vi "Event Handler.vi"(0 "Tamer in":refnum<class "Tamer.lvclass">, 5 "Event type":T1=enum."Message", 7 "Item Name":string, 9 "Data":variant, 11 "error in (no error)":errorcluster) -> (4 "Tamer out":refnum<class "Tamer.lvclass">, 15 "error out":errorcluster)   [LabVIEW 2020, in "Tamer.lvlib" / "Tamer.lvclass"]
doc: "This VI is the event handler of the uService: every time an event is triggered to the uService, this VI is called.\nNote: here you can access the Actor/Class data, but it will be the one coming out from Init. You cannot modify the values.\nThree different events are supported:\nI) Button Pressed: get called on a GUI button pressed. Item Name is the name (label) of the button, Data is empty.\nII) Shared Variable Updated: get called when a SV you subscribed to is updated. Item Name is the name of the SV, and Data is the value (note: you need to convert it to the proper type).\nIII) Message: get called every time a user event is generated using Send Message to Event Handler. The values of Item Name and Data are the one given to the Send Message to Event Handler.\nIV) Ready to launch?: this frame get called every time a new Run is initiated. Each uService is responsible of performing a self check before giving back the green light for the Run to start."
uses:
  Tamer.lvclass
  C:/Users/marco/Documents/GitHub_Lab/TALOS/talos/Father of all uServices/Father of all uServices/Father of all uServices.lvclass
  Father of all uServices/Father of all uServices/Event Handler Items.ctl
  Ancestor/Ancestor/Ancestor.lvclass/Ancestor.ctl
  Tamer Consumer Case Selector.ctl
  Father of all uServices/Father of all uServices Messages/Consumer Msg/Consumer Msg.lvclass/Consumer Msg.ctl
  Support VIs/Go-NoGo.ctl
  Run Utilities/TypeDefs/Messages/Monkey Status Message.ctl
  Run Utilities/TypeDefs/Monkey Status.ctl
  Run Utilities/Schedule/Schedule.lvclass
  Run Utilities/TypeDefs/Messages/Script Checker Message.ctl
  Run Utilities/TypeDefs/Script Checker Result.ctl
  Run Utilities/TypeDefs/Messages/Banana Message.ctl
  Run Utilities/TypeDefs/Return Code.ctl
  Guardian/Guardian Messages/Message to uService Msg/Message to uService Msg.lvclass/Message to uService Msg.ctl
  Tamer.lvclass/Tamer.ctl
  Guardian/Guardian/Requests.ctl
  Guardian/Guardian Messages/Requests from uServices Msg/Requests from uServices Msg.lvclass/Requests from uServices Msg.ctl
  FGV/Error Memory/Get Error Description.vi
  Support VIs/Get PC name.vi
  Ancestor/Ancestor/Read ID.vi
  Support VIs/Get Class Name.vi
  <vilib>/Utility/error.llb/Clear Errors.vi
  Father of all uServices/Father of all uServices Messages/Consumer Msg/Send Consumer.vi
  Guardian/Guardian Messages/Message to uService Msg/Send Message to uService.vi
  Guardian/Guardian Messages/Requests from uServices Msg/Send Requests from uServices.vi
  FGV/Error Memory/Error Memory Core.vi
  <vilib>/AdvancedString/Delimited String to 1D String Array.vi
  Support VIs/Circus Root Path.vi
  FGV/Error Memory/Error Crt Lvl checker.vi
  FGV/Error Memory/Error Memory Core.vi/40c8088d-b597-4017-91af-faa98e00292e.vi
  FGV/Error Memory/Error Memory Core.vi/d4a3ab98-063c-4e44-b43d-fbdcfe6c2be2.vi
  Father of all uServices/Father of all uServices/Father of all uServices.lvclass
  C:/Users/marco/Documents/GitHub_Lab/TALOS/builds/Actor Framework PPL/Actor Framework.lvlibp/1abvi3w/vi.lib/ActorFramework/Actor/Actor.lvclass
  Support VIs/Global Memory.vi
  <vilib>/Utility/LVClass/Get LV Class Name.vi
  Support VIs/Is in Packed Library.vi
  Support VIs/TALOS Root path.vi
  Support VIs/Read CSV worksheet.vi
  Support VIs/Global Constants.vi
  <vilib>/Utility/error.llb/General Error Handler.vi
  builds/Actor Framework PPL/Actor Framework.lvlibp/1abvi3w/vi.lib/ActorFramework/Actor/Read Self Enqueuer.vi
  <userlib>/_OpenG.lib/lvdata/lvdata.llb/Get Strings from Enum__ogtk.vi
  builds/Actor Framework PPL/Actor Framework.lvlibp/1abvi3w/vi.lib/ActorFramework/Message Enqueuer/Enqueue.vi
  Support VIs/Error Log.vi
  Open Debug Window.vi
  builds/Actor Framework PPL/Actor Framework.lvlibp/1abvi3w/vi.lib/ActorFramework/Actor/Read Caller Enqueuer.vi
  Ancestor/Ancestor/Ancestor.lvclass
  <vilib>/Comparison/Equal/Equal Functor/Equal Functor.lvclass
  Father of all uServices/Father of all uServices Messages/Consumer Msg/Consumer Msg.lvclass
  Guardian/Guardian Messages/Message to uService Msg/Message to uService Msg.lvclass
  Guardian/Guardian Messages/Requests from uServices Msg/Requests from uServices Msg.lvclass
  TALOS.lvlib
  Guardian/Guardian/Guardian.lvclass
  Run Utilities/Run Utilities.lvlib
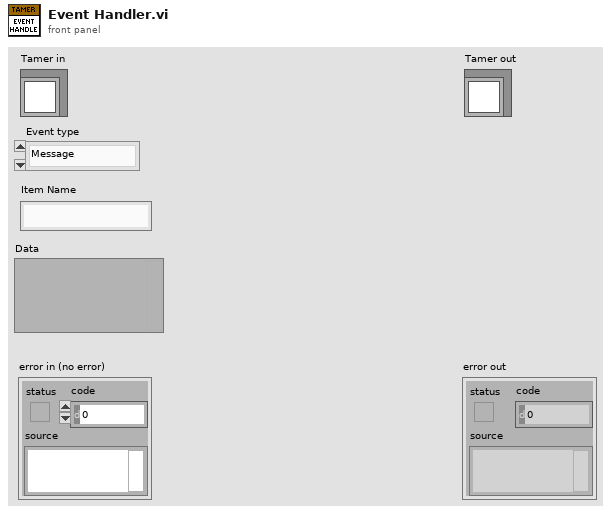
[diagram p1: front panel]
types:
  T1 = typedef "TALOS.lvlib/Father of all uServices.lvlib/Father of all uServices.lvclass/Event Handler Items.ctl" = enum16{"Button Pressed", "Shared Variable Updated", "Message", "Ready to launch?", "Safe Mode", "Start RUN", "Stop RUN"}
  T2 = typedef "Tamer.lvlib/Tamer.lvclass/Tamer Consumer Case Selector.ctl" = enum16{"New schedule", "Initiate RUN", "Parse Schedules", "Script Checker", "Banana after Quality Check", "Update Crit Lvl", "Propagate Banana", "Reply from Guardian", "Reply from uService", "Timeout of RUN", "uService Replies Check", "Update from Monkey", "Monkey Died", "Reschedule", "Rerun", "Stop DAQ", "Stop Schedule", "Skip Run", "Kill Process", "Update GV"}
  T3 = enum32{"Invalid", "Standard", "Closed", "Hidden", "Minimized", "Maximized"}
  T4 = typedef "TALOS.lvlib/Go-NoGo.ctl" = cluster{"ID":string, "Status":bool, "Data":string[], "GUID":string}
  T5 = typedef "TALOS.lvlib/Run Utilities.lvlib/Monkey Status Message.ctl" = cluster{"Monkey ID":string, "Monkey Status":T6, "Scripts left":u32, "ETA":string, "Current Action":string, "Report from previous RUNs":string, "Skipped RUNs":refnum<class "Schedule.lvclass">}
  T6 = typedef "TALOS.lvlib/Run Utilities.lvlib/Monkey Status.ctl" = enum16{"Init", "Paused", "Ongoing", "Stopped", "Finished (no errors)", "Finished (with errors)"}
  T7 = typedef "TALOS.lvlib/Run Utilities.lvlib/Script Checker Message.ctl" = cluster{"Monkey ID":string, "Script Checker Result":T8}
  T8 = typedef "TALOS.lvlib/Run Utilities.lvlib/Script Checker Result.ctl" = enum16{"Passed", "Failed", "Empty"}
  T9 = typedef "TALOS.lvlib/Run Utilities.lvlib/Return Code.ctl" = enum16{"All Good", "Retry", "Skip", "Skip All", "ABORT"}
  T10 = typedef "TALOS.lvlib/Run Utilities.lvlib/Banana Message.ctl" = cluster{"FPGA Name":string, "Return Code":T9}
  T11 = typedef "TALOS.lvlib/Guardian.lvlib/Guardian.lvclass/Requests.ctl" = enum16{"Ready to Launch", "Start RUN", "Stop RUN", "Update DAQ Params", "Update Error Listbox", "Update Run Status", "Update Kasli Log", "Run Stopped with Errors", "Switch uS View"}
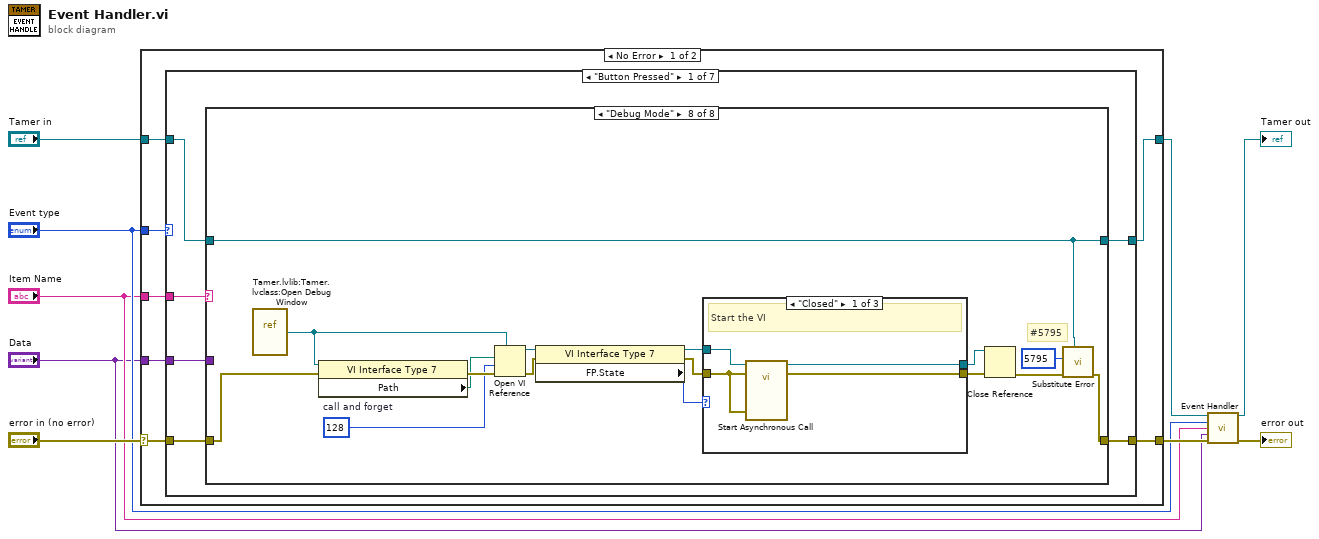
[diagram p0: block diagram]
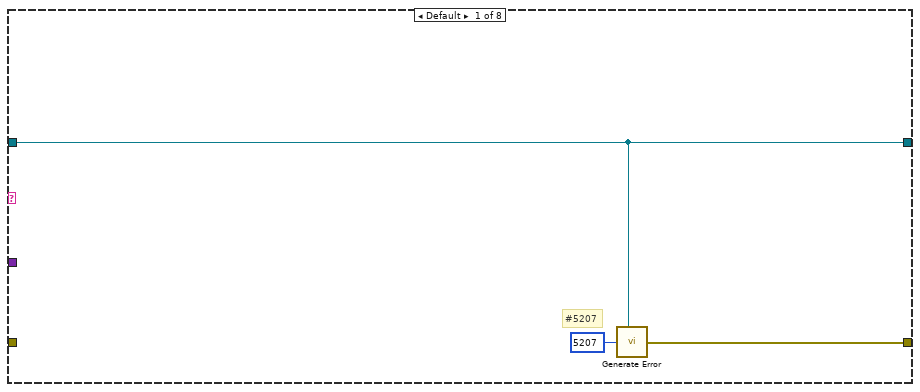
[diagram p2: hidden frame]
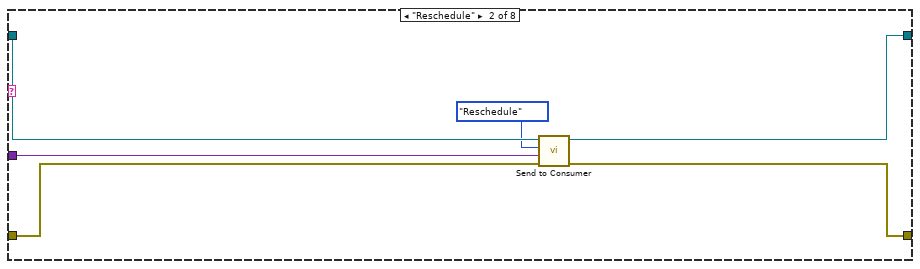
[diagram p3: hidden frame]
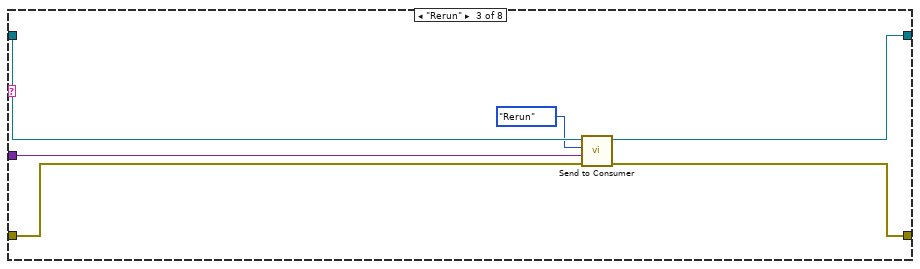
[diagram p4: hidden frame]
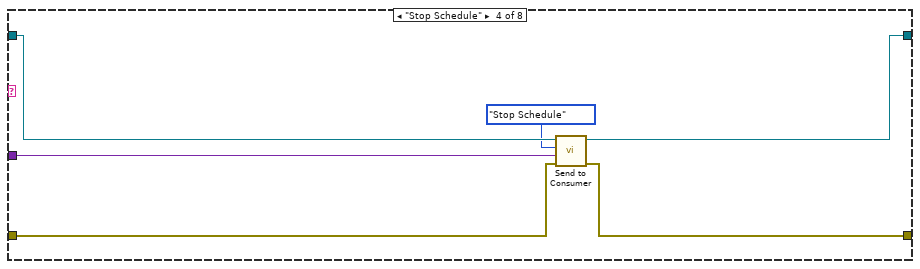
[diagram p5: hidden frame]
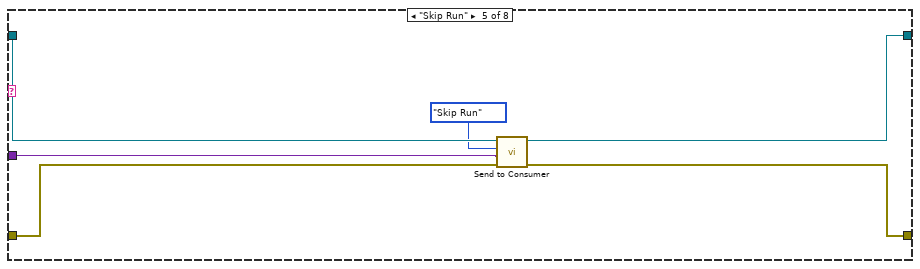
[diagram p6: hidden frame]
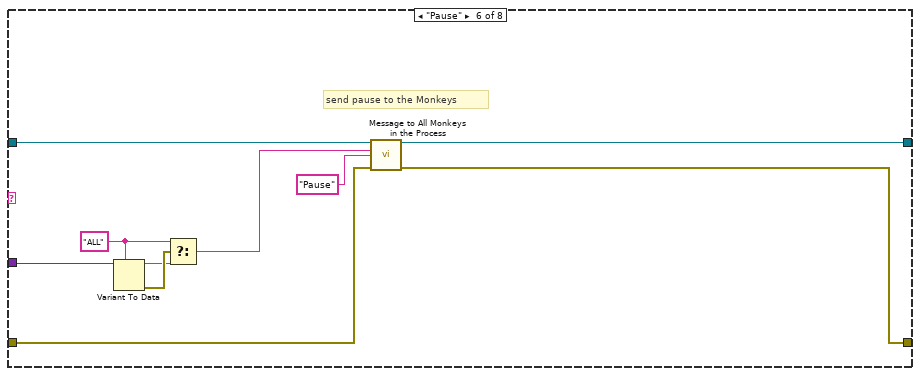
[diagram p7: hidden frame]
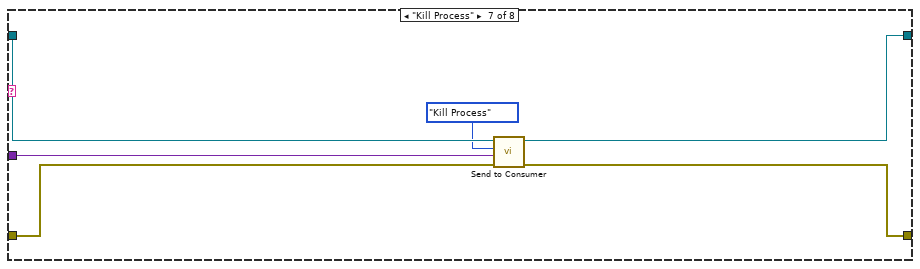
[diagram p8: hidden frame]
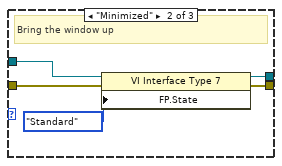
[diagram p9: hidden frame]
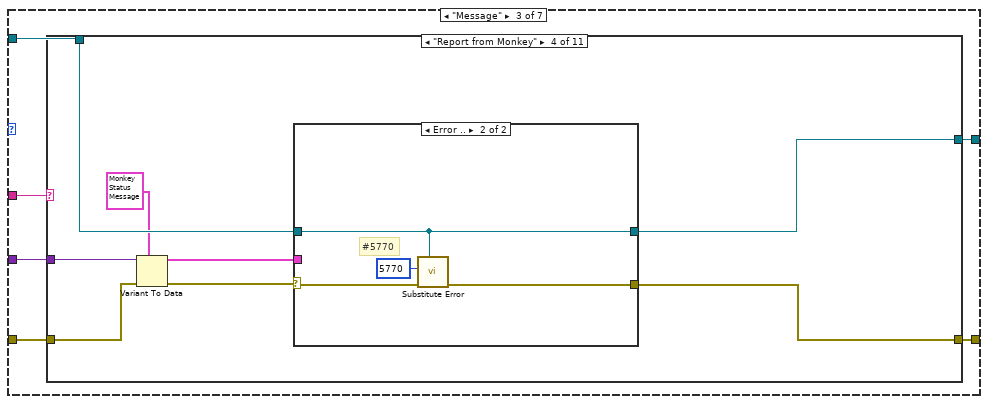
[diagram p12: hidden frame]
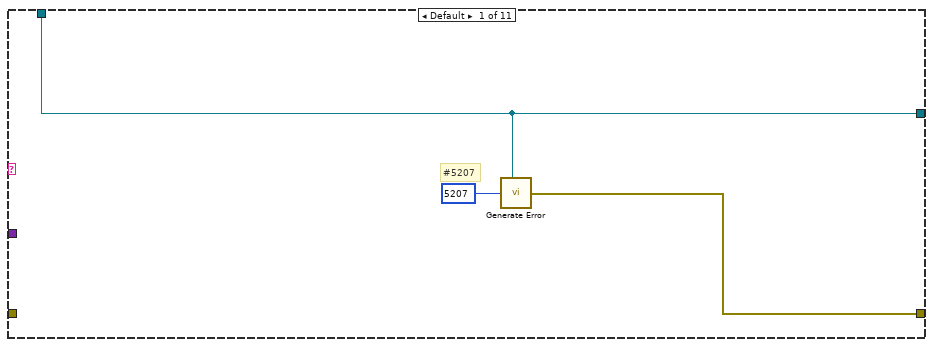
[diagram p13: hidden frame]
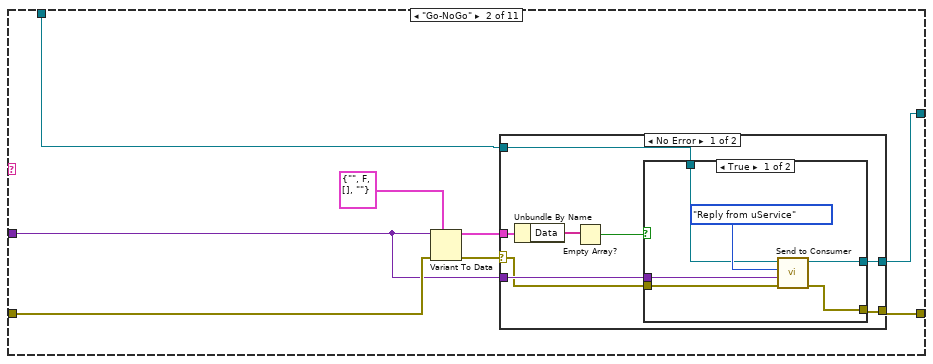
[diagram p14: hidden frame]
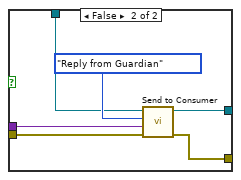
[diagram p15: hidden frame]
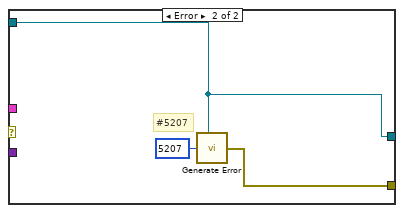
[diagram p16: hidden frame]
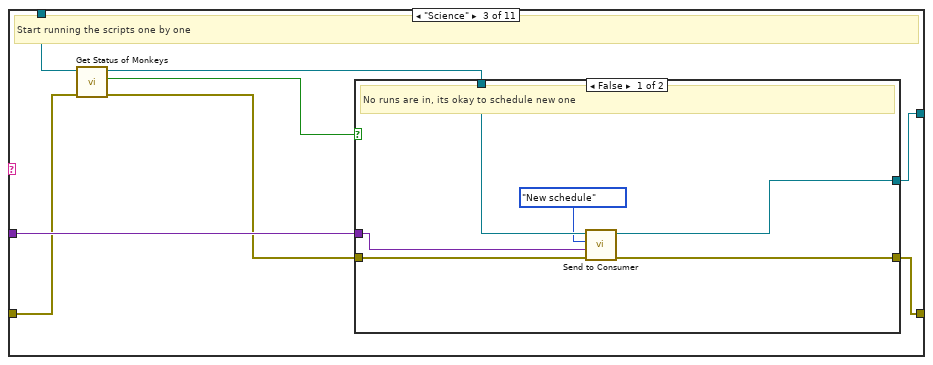
[diagram p17: hidden frame]
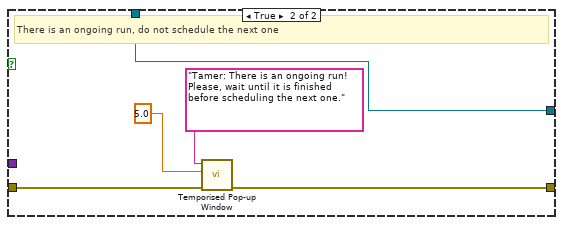
[diagram p18: hidden frame]
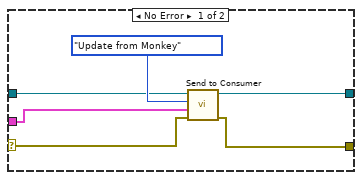
[diagram p19: hidden frame]
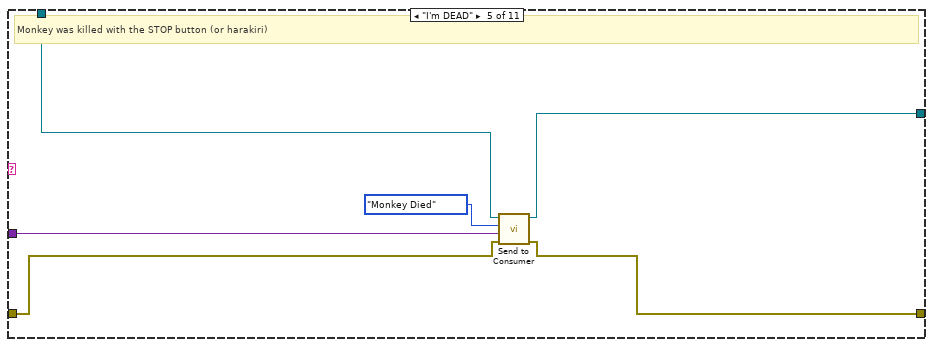
[diagram p20: hidden frame]
diagram:
  n1 = case shown="No Error" "error in (no error)" {
    selector: "error in (no error)" -> [w14 w330]
    tunnel: [w15 w330] -> w7
    tunnel: [w11 w329] -> w4
    tunnel: "Tamer in" -> [w10 w329]
    tunnel: "Event type" -> [w16 _]
    tunnel: "Item Name" -> [w13 _]
    tunnel: "Data" -> [w12 _]
    frame No Error {
      n2 = case shown="\"Button Pressed\"" w16 {
        tunnel: [w22 w94 w96 w307 w316 w321 w328] -> w15
        tunnel: w14 -> [w19 w94 w100 w308 w318 w322 w326]
        tunnel: w13 -> [w20 _ w99 _ _ _ _]
        tunnel: w10 -> [w21 w93 w97 w306 w313 w323 w327]
        tunnel: w12 -> [w17 _ w98 w304 _ _ _]
        tunnel: [w18 w93 w95 w303 w315 w319 w324] -> w11
        frame "Button Pressed" {
          n3 = case shown="\"Debug Mode\"" w20 {
            tunnel: w19 -> [_ w26 w32 w39 w45 w56 w63 w77]
            tunnel: [w24 w30 w35 w42 w46 w55 w60 w66] -> w22
            tunnel: w21 -> [w23 w31 w37 w43 w49 w58 w65 w67]
            tunnel: [w23 w28 w34 w41 w47 w57 w61 w67] -> w18
            tunnel: w17 -> [_ w27 w33 w38 w44 w54 w62 _]
            frame Default {
              # "#5207"
              n4 = call "Generate Error.vi"("Class"=w23, "Error Code"=5207) -> ("error out"=w24:errorcluster)  [unwired: 5 in]
            }
            frame "Reschedule" {
              n5 = call "Send to Consumer.vi"("error in (no error)"=w26, "Data"=w27, "Case ID"=Tamer_Consumer_Case_Selector."Reschedule" ("Monkey Consumer Case Selector"), "uService Template in"=w31) -> ("error out"=w30:errorcluster, "uService Template out"=w28:refnum<class "Tamer.lvclass">)  [unwired: 6 in]
            }
            frame "Rerun" {
              n6 = call "Send to Consumer.vi"("error in (no error)"=w32, "Data"=w33, "Case ID"=Tamer_Consumer_Case_Selector."Rerun" ("Monkey Consumer Case Selector"), "uService Template in"=w37) -> ("error out"=w35:errorcluster, "uService Template out"=w34:refnum<class "Tamer.lvclass">)  [unwired: 6 in]
            }
            frame "Stop Schedule" {
              n7 = call "Send to Consumer.vi"("error in (no error)"=w39, "Data"=w38, "Case ID"=Tamer_Consumer_Case_Selector."Stop Schedule" ("Monkey Consumer Case Selector"), "uService Template in"=w43) -> ("error out"=w42:errorcluster, "uService Template out"=w41:refnum<class "Tamer.lvclass">)  [unwired: 6 in]
            }
            frame "Skip Run" {
              n8 = call "Send to Consumer.vi"("error in (no error)"=w45, "Data"=w44, "Case ID"=Tamer_Consumer_Case_Selector."Skip Run" ("Monkey Consumer Case Selector"), "uService Template in"=w49) -> ("error out"=w46:errorcluster, "uService Template out"=w47:refnum<class "Tamer.lvclass">)  [unwired: 6 in]
            }
            frame "Pause" {
              w53 = "ALL"
              # "send pause to the Monkeys"
              n9 = Variant To Data(type=w53, Variant=w54) -> (data=w52:string, error out=w59:errorcluster)  [unwired: 1 in]
              n10 = Select(t=w53, s=w59, f=w52) -> (s? t:f=w51:string)
              n11 = call-dynamic "Message to All Monkeys in the Process.vi"("Tamer in"=w58, "Process ID"=w51, "Message"="Pause" ("Process ID"), "error in (no error)"=w56) -> ("Tamer out"=w57:refnum<class "Tamer.lvclass">, "error out"=w55:errorcluster)  [unwired: 10 in]
            }
            frame "Kill Process" {
              n12 = call "Send to Consumer.vi"("error in (no error)"=w63, "Data"=w62, "Case ID"=Tamer_Consumer_Case_Selector."Kill Process" ("Monkey Consumer Case Selector"), "uService Template in"=w65) -> ("error out"=w60:errorcluster, "uService Template out"=w61:refnum<class "Tamer.lvclass">)  [unwired: 6 in]
            }
            frame "Debug Mode" {
              w78 = 128  # call and forget
              # "#5795"
              n13 = vi-ref "Tamer.lvlib:Tamer.lvclass:Open Debug Window.vi"() -> (w76:refnum<vi>)
              n14 = property class="VI Interface Type 7"(reference=w76, error in=w77) -> (error out=w81:errorcluster, "Path"=w80:path)  [unwired: 1 out]
              n15 = Open VI Reference(type specifier VI Refnum (for type only)=w76, vi path=w80, options=w78, error in (no error)=w81) -> (vi reference=w79:refnum<vi>, error out=w74:errorcluster)  [unwired: 2 in]
              n16 = property class="VI Interface Type 7"(reference=w79, error in=w74) -> (reference out=w75:refnum<vi>, error out=w73:errorcluster, "FP.State"=w72:T3)
              n17 = case shown="\"Closed\"" w72 {
                tunnel: w75 -> [w85 w88 w92]
                tunnel: w73 -> [w84 w90 w91]
                tunnel: [w83 w89 w91] -> w69
                tunnel: [w82 w86 w92] -> w68
                frame "Closed" {
                  # "Start the VI"
                  n18 = call-by-ref "Start Asynchronous Call"(reference=w85, error in=w84, 8:"error in (no error)"=w84) -> (reference out=w82:refnum<vi>, error out=w83:errorcluster)  [unwired: 10 in, 1 out]
                }
                frame "Minimized" {
                  # "Bring the window up"
                  n19 = property class="VI Interface Type 7"(reference=w88, error in=w90, "FP.State"=T3."Standard" ("Front Panel Window:State")) -> (reference out=w86:refnum<vi>, error out=w89:errorcluster)
                }
                frame Default {
                  # "Either running or something is worng, do nothing"
                }
              }
              n20 = Close Reference(reference=w68, error in (no error)=w69) -> (error out=w71:errorcluster)
              n21 = call "Substitute Error.vi"("LabVIEW Object"=w67, "error in (no error)"=w71, "Error Code"=5795) -> ("error out"=w66:errorcluster)  [unwired: 8 in]
            }
          }
        }
        frame "Shared Variable Updated" {
        }
        frame "Message" {
          n22 = case shown="\"Report from Monkey\"" w99 {
            tunnel: w100 -> [_ w110 w140 w160 w173 w184 w201 w239 w259 w276 w293]
            tunnel: w98 -> [_ w107 w142 w161 w174 w183 w203 w235 w258 w281 _]
            tunnel: w97 -> [w101 w105 w139 w158 w177 w180 w197 w240 w257 w278 w290]
            tunnel: [w102 w111 w141 w155 w176 w178 w198 w236 w260 w271 w292] -> w96
            tunnel: [w101 w104 w135 w154 w172 w179 w196 w245 w256 w279 w291] -> w95
            frame Default {
              # "#5207"
              n23 = call "Generate Error.vi"("Class"=w101, "Error Code"=5207) -> ("error out"=w102:errorcluster)  [unwired: 5 in]
            }
            frame "Go-NoGo" {
              n24 = Variant To Data(error in=w110, type=T4 {"ID"="", "Status"=FALSE, "Data"=[], "GUID"=""} ("Go-NoGo"), Variant=w107) -> (data=w106:T4, error out=w108:errorcluster)
              n25 = case shown="No Error" w108 {
                selector: w108 -> [w114 _]
                tunnel: [w119 w133] -> w111
                tunnel: w107 -> [w118 _]
                tunnel: w106 -> [w117 _]
                tunnel: w105 -> [w113 w132]
                tunnel: [w112 w132] -> w104
                frame No Error {
                  n26 = Unbundle By Name(w117) -> ("Data"=w116:string[])
                  n27 = Empty Array?(array=w116) -> (empty?=w115:bool)
                  n28 = case shown="True" w115 {
                    tunnel: [w125 w131] -> w119
                    tunnel: w118 -> [w123 w129]
                    tunnel: w114 -> [w122 w128]
                    tunnel: w113 -> [w121 w127]
                    tunnel: [w120 w126] -> w112
                    frame True {
                      n29 = call "Send to Consumer.vi"("error in (no error)"=w122, "Data"=w123, "Case ID"=Tamer_Consumer_Case_Selector."Reply from uService" ("Monkey Consumer Case Selector"), "uService Template in"=w121) -> ("error out"=w125:errorcluster, "uService Template out"=w120:refnum<class "Tamer.lvclass">)  [unwired: 6 in]
                    }
                    frame False {
                      n30 = call "Send to Consumer.vi"("error in (no error)"=w128, "Data"=w129, "Case ID"=Tamer_Consumer_Case_Selector."Reply from Guardian" ("Monkey Consumer Case Selector"), "uService Template in"=w127) -> ("error out"=w131:errorcluster, "uService Template out"=w126:refnum<class "Tamer.lvclass">)  [unwired: 6 in]
                    }
                  }
                }
                frame Error {
                  # "#5207"
                  n31 = call "Generate Error.vi"("Class"=w132, "Error Code"=5207) -> ("error out"=w133:errorcluster)  [unwired: 5 in]
                }
              }
            }
            frame "Science" {
              # "Start running the scripts one by one"
              n32 = call-dynamic "Get Status of Monkeys.vi"("error in (no error)"=w140, "Tamer in"=w139) -> ("error out"=w137:errorcluster, "Anything running?"=w136:bool, "Tamer out"=w138:refnum<class "Tamer.lvclass">)  [unwired: 7 in]
              n33 = case shown="False" w136 {
                tunnel: w142 -> [w145 _]
                tunnel: [w148 w150] -> w141
                tunnel: w138 -> [w147 w149]
                tunnel: w137 -> [w144 w153]
                tunnel: [w143 w149] -> w135
                frame False {
                  # "No runs are in, its okay to schedule new one"
                  n34 = call "Send to Consumer.vi"("error in (no error)"=w144, "Data"=w145, "Case ID"=Tamer_Consumer_Case_Selector."New schedule" ("Monkey Consumer Case Selector"), "uService Template in"=w147) -> ("error out"=w148:errorcluster, "uService Template out"=w143:refnum<class "Tamer.lvclass">)  [unwired: 6 in]
                }
                frame True {
                  # "There is an ongoing run, do not schedule the next one"
                  n35 = call "Temporised Pop-up Window.vi"("error in (no error)"=w153, "Timeout"=5.0, "Text"="Tamer: There is an ongoing run! Please, wait until it is finished before scheduling the next one.") -> ("error out"=w150:errorcluster)  [unwired: 8 in]
                }
              }
            }
            frame "Report from Monkey" {
              n36 = Variant To Data(error in=w160, type=T5 {"Monkey ID"="", "Monkey Status"=enum."Ongoing", "Scripts left"=0, "ETA"="", "Current Action"="", "Report from previous RUNs"="", "Skipped RUNs"=refnum} ("Monkey Status Message"), Variant=w161) -> (data=w157:T5, error out=w159:errorcluster)
              n37 = case shown="Error .." w159 {
                selector: w159 -> [w166 w171]
                tunnel: w158 -> [w165 w168]
                tunnel: w157 -> [w164 _]
                tunnel: [w163 w169] -> w155
                tunnel: [w162 w168] -> w154
                frame No Error {
                  n38 = call "Send to Consumer.vi"("error in (no error)"=w166, "Data"=w164, "Case ID"=Tamer_Consumer_Case_Selector."Update from Monkey" ("Monkey Consumer Case Selector"), "uService Template in"=w165) -> ("error out"=w163:errorcluster, "uService Template out"=w162:refnum<class "Tamer.lvclass">)  [unwired: 6 in]
                }
                frame Error {
                  # "#5770"
                  n39 = call "Substitute Error.vi"("LabVIEW Object"=w168, "error in (no error)"=w171, "Error Code"=5770) -> ("error out"=w169:errorcluster)  [unwired: 8 in]
                }
              }
            }
            frame "I'm DEAD" {
              # "Monkey was killed with the STOP button (or harakiri)"
              n40 = call "Send to Consumer.vi"("error in (no error)"=w173, "Data"=w174, "Case ID"=Tamer_Consumer_Case_Selector."Monkey Died" ("Monkey Consumer Case Selector"), "uService Template in"=w177) -> ("error out"=w176:errorcluster, "uService Template out"=w172:refnum<class "Tamer.lvclass">)  [unwired: 6 in]
            }
            frame "Script Checker" {
              # "Synced Monkey Performed Script Check"
              n41 = Variant To Data(error in=w184, type=T7 {"Monkey ID"="", "Script Checker Result"=enum."Passed"} ("Message"), Variant=w183) -> (data=w181:T7, error out=w182:errorcluster)
              n42 = case shown="Error .." w182 {
                selector: w182 -> [w187 w193]
                tunnel: [w191 w194] -> w178
                tunnel: w180 -> [w190 w192]
                tunnel: w181 -> [w189 _]
                tunnel: [w186 w192] -> w179
                frame No Error {
                  n43 = call "Send to Consumer.vi"("error in (no error)"=w187, "Data"=w189, "Case ID"=Tamer_Consumer_Case_Selector."Script Checker" ("Monkey Consumer Case Selector"), "uService Template in"=w190) -> ("error out"=w191:errorcluster, "uService Template out"=w186:refnum<class "Tamer.lvclass">)  [unwired: 6 in]
                }
                frame Error {
                  # "#5757"
                  n44 = call "Substitute Error.vi"("LabVIEW Object"=w192, "error in (no error)"=w193, "Error Code"=5757) -> ("error out"=w194:errorcluster)  [unwired: 8 in]
                }
              }
            }
            frame "B4n4n4" {
              # "Script finished. Send it to Monkey for the quality check"
              n45 = Variant To Data(error in=w201, type=string[] [], Variant=w203) -> (data=w200:string[], error out=w199:errorcluster)
              n46 = case shown="No Error" w199 {
                selector: w199 -> [w226 w234]
                tunnel: w200 -> [w230 _]
                tunnel: [w210 w233] -> w198
                tunnel: w197 -> [w224 w231]
                tunnel: [w221 w231] -> w196
                frame No Error {
                  w204 = "Quality Check" ("Message")
                  # "#5752\nB4n4n4"
                  n47 = Index Array(array=w230) -> (element #1=w211:string, element #2=w227:string)  [unwired: 2 in]
                  n48 = Decimal String To Number(string=w227, default (0L)=3) -> (number=w228:i32)  [unwired: 1 in, 1 out]
                  n49 = Variant To Data(error in=w226, type=Return_Code."Skip All" ("Return Code"), Variant=w228) -> (data=w220:T9, error out=w223:errorcluster)
                  n50 = call-dynamic "Get Monkey ID From FPGA Name.vi"("error in (no error)"=w223, "FPGA Name"=w211, "Tamer in"=w224) -> ("error out"=w219:errorcluster, "Monkey ID"=w214:string, "Tamer out"=w218:refnum<class "Tamer.lvclass">)  [unwired: 6 in]
                  n51 = Bundle(cluster=T10 {"FPGA Name"="", "Return Code"=enum."All Good"} ("Cluster"), "FPGA Name"=w211, "Return Code"=w220) -> (w209:T10)
                  n52 = call "Message to uService.vi"("Father of all uServices in"=w218, "uService ID"=w214, "Message"=w204, "Data"=w209, "error in (no error)"=w219) -> ("Father of all uServices out"=w208:refnum<class "Tamer.lvclass">, "error out"=w215:errorcluster)  [unwired: 9 in]
                  n53 = Concatenate Strings(w204, " to " ("string"), w214) -> (w213:string)
                  n54 = call "FPGA informative error on return.vi"("Message"=w209, "Class in"=w208) -> ("error out"=w206:errorcluster)  [unwired: 9 in]
                  n55 = call-dynamic "Update Action History.vi"("error in (no error)"=w215, "Action"=w213, "Tamer in"=w208) -> ("error out"=w207:errorcluster, "Tamer out"=w221:refnum<class "Tamer.lvclass">)  [unwired: 7 in]
                  n56 = Merge Errors(w207, w206) -> (w205:errorcluster)
                  n57 = call "Substitute Error.vi"("LabVIEW Object"=w221, "error in (no error)"=w205, "Error Code"=5752, "Optional String"="Tamer doesn't know who sent B4n4n4") -> ("error out"=w210:errorcluster)  [unwired: 7 in]
                }
                frame Error {
                  # "#5789"
                  n58 = call "Substitute Error.vi"("LabVIEW Object"=w231, "error in (no error)"=w234, "Error Code"=5789) -> ("error out"=w233:errorcluster)  [unwired: 8 in]
                }
              }
            }
            frame "Quality Check - result" {
              n59 = Variant To Data(type=T10 {"FPGA Name"="", "Return Code"=enum."All Good"} ("Cluster"), Variant=w235) -> (data=w241:T10, error out=w242:errorcluster)  [unwired: 1 in]
              n60 = case shown="No Error" w242 {
                tunnel: w241 -> [w250 _]
                tunnel: w240 -> [w253 w254]
                tunnel: [w248 _] -> w237
                tunnel: [w249 w254] -> w246
                frame No Error {
                  # "Check if quality of run was passed. If not, give an error to have that information in the error log"
                  n61 = Unbundle By Name(w250) -> ("FPGA Name"=w251:string)
                  n62 = Concatenate Strings("Received the quality check from ", w251) -> (w247:string)
                  n63 = call-dynamic "Update Action History.vi"("Action"=w247, "Tamer in"=w253) -> ("error out"=w248:errorcluster, "Tamer out"=w249:refnum<class "Tamer.lvclass">)  [unwired: 8 in]
                }
                frame Error {
                  # "Wrong format, this is delt with in the consumer"
                }
              }
              n64 = call "Send to Consumer.vi"("error in (no error)"=w239, "Data"=w235, "Case ID"=Tamer_Consumer_Case_Selector."Banana after Quality Check" ("Monkey Consumer Case Selector"), "uService Template in"=w246) -> ("error out"=w238:errorcluster, "uService Template out"=w245:refnum<class "Tamer.lvclass">)  [unwired: 6 in]
              n65 = Merge Errors(w238, w237) -> (w236:errorcluster)
            }
            frame "570prun" {
              # "True= StartRun given, False = StopRun given"
              # "Issue Stop Run to all the uServices and Guardians."
              n66 = Unbundle By Name(w257) -> ("StartRun/StopRun toggle"=w255:bool)
              n67 = case shown="True" w255 {
                tunnel: [w262 w270] -> w260
                tunnel: w259 -> [w262 w269]
                tunnel: w258 -> [_ w268]
                tunnel: w257 -> [w261 w266]
                tunnel: [w261 w264] -> w256
                frame False {
                  # "Do nothing"
                }
                frame True {
                  # "#STOP_RUN"
                  n68 = call "Request to Guardian.vi"("error in (no error)"=w269, "Data"=w268, "Requests"=Requests."Stop RUN", "Father of all uServices in"=w266) -> ("error out"=w270:errorcluster, "Father of all uServices out"=w265:refnum<class "Tamer.lvclass">)  [unwired: 6 in]
                  n69 = Bundle By Name(cluster=w265, "StartRun/StopRun toggle"=FALSE) -> (w264:refnum<class "Tamer.lvclass">)
                }
              }
            }
            frame "Error Criticality" {
              # "Error occured when running a script"
              n70 = call-dynamic "Get Status of Monkeys.vi"("error in (no error)"=w276, "Tamer in"=w278) -> ("error out"=w282:errorcluster, "Anything running?"=w274:bool, "Tamer out"=w277:refnum<class "Tamer.lvclass">)  [unwired: 7 in]
              n71 = Not(x=w282) -> (.not. x?=w275:bool)
              n72 = Select(t=w274, s=w275, f=TRUE) -> (s? t:f=w272:bool)
              n73 = case shown="True" w272 {
                tunnel: w281 -> [_ w287]
                tunnel: [_ w286] -> w280
                tunnel: [w283 w284] -> w279
                tunnel: w277 -> [w283 w288]
                frame False {
                }
                frame True {
                  n74 = call "Send to Consumer.vi"("Data"=w287, "Case ID"=Tamer_Consumer_Case_Selector."Update Crit Lvl" ("Monkey Consumer Case Selector"), "uService Template in"=w288) -> ("error out"=w286:errorcluster, "uService Template out"=w284:refnum<class "Tamer.lvclass">)  [unwired: 7 in]
                }
              }
              n75 = Merge Errors(w280, w282) -> (w271:errorcluster)
            }
            frame "5cr47ch_y0ur_h34d" {
              # "True= StartRun given, False = StopRun given"
              # "Start the Run, but only if wasn't already started"
              n76 = Unbundle By Name(w290) -> ("StartRun/StopRun toggle"=w289:bool)
              n77 = case shown="False" w289 {
                tunnel: w293 -> [w300 w301]
                tunnel: [w299 w301] -> w292
                tunnel: [w296 w302] -> w291
                tunnel: w290 -> [w294 w302]
                frame False {
                  # "#START_RUN"
                  n78 = call "Request to Guardian.vi"("error in (no error)"=w300, "Requests"=Requests."Start RUN", "Father of all uServices in"=w294) -> ("error out"=w299:errorcluster, "Father of all uServices out"=w298:refnum<class "Tamer.lvclass">)  [unwired: 7 in]
                  n79 = Bundle By Name(cluster=w298, "StartRun/StopRun toggle"=TRUE ("StartRun already given?")) -> (w296:refnum<class "Tamer.lvclass">)
                }
                frame True {
                  # "Do nothing"
                }
              }
            }
          }
        }
        frame "Ready to launch?" {
          # "Don't remove this wire!"
          # "Just give green light: \"Cogito ergo sum\" - Volpe"
          n80 = call-dynamic "Go-NoGo.vi"("error in (no error)"=w308, "Go-NoGo Data"=w304, "Go?"=TRUE, "Father of all uServices in"=w306) -> ("error out"=w307:errorcluster, "Father of all uServices out"=w303:refnum<class "Tamer.lvclass">)  [unwired: 6 in]
        }
        frame "Safe Mode" {
          n81 = call-dynamic "Update Monkeys Status.vi"("In ALL?"=TRUE, "Status"=Monkey_Status."Finished (with errors)", "Tamer in"=w313) -> ("error out"=w311:errorcluster, "Tamer out"=w314:refnum<class "Tamer.lvclass">)  [unwired: 7 in]
          n82 = call "Send to Consumer.vi"("Case ID"=Tamer_Consumer_Case_Selector."Stop Schedule" ("Monkey Consumer Case Selector"), "uService Template in"=w314) -> ("error out"=w312:errorcluster, "uService Template out"=w315:refnum<class "Tamer.lvclass">)  [unwired: 8 in]
          n83 = Merge Errors(w312, w311, w318) -> (w316:errorcluster)
        }
        frame "Start RUN" {
          n84 = call-dynamic "Update Action History.vi"("error in (no error)"=w322, "Action"="Start Run" ("GUI Item Name"), "Tamer in"=w323) -> ("error out"=w321:errorcluster, "Tamer out"=w319:refnum<class "Tamer.lvclass">)  [unwired: 7 in]
        }
        frame "Stop RUN" {
          n85 = call-dynamic "Update Action History.vi"("error in (no error)"=w326, "Action"="Experiment finished! Ending the script..." ("GUI Item Name"), "Tamer in"=w327) -> ("error out"=w328:errorcluster, "Tamer out"=w324:refnum<class "Tamer.lvclass">)  [unwired: 7 in]
        }
      }
    }
    frame Error {
    }
  }
  n86 = call-parent "Event Handler.vi"("uService Template in"=w4, "Event type"="Event type", "Item Name"="Item Name", "Data"="Data", "error in (no error)"=w7) -> ("uService Template out"=→"Tamer out":refnum<class "Tamer.lvclass">, "error out"=→"error out":errorcluster)  [unwired: 9 in]
